vi "Update Block Status.vi"(4 "Writing":bool, 6 "Working":bool, 8 "Worker Error":errorcluster, 9 "Status In":T1={"State"=enum."Init", "i"=0, "Init"=FALSE, "Started"=FALSE, "Action"=enum."N/A"}, 11 "Status Queue In":refnum<queue>) -> (1 "Status":T1={"State"=enum."Init", "i"=0, "Init"=FALSE, "Started"=FALSE, "Action"=enum."N/A"}, 3 "Status Queue":refnum<queue>)   [LabVIEW 2020, in "FlexBlocks.lvlib"]
uses:
  FlexBlocks.lvlib
  Block Status.ctl
  Block State.ctl
  Run Action.ctl
  Block Status with Error.ctl
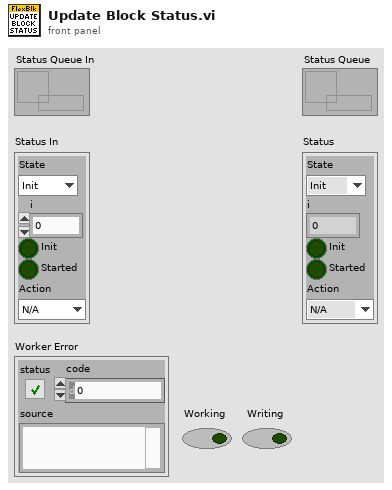
[diagram p1: front panel]
types:
  T1 = typedef "FlexBlocks.lvlib/Block Status.ctl" = cluster{"State":T2, "i":i32, "Init":bool, "Started":bool, "Action":T3}
  T2 = typedef "FlexBlocks.lvlib/Block State.ctl" = enum16{"Idle", "Init", "Start", "Run", "Stop"}
  T3 = typedef "FlexBlocks.lvlib/Run Action.ctl" = enum16{"N/A", "Read", "Work", "Write"}
  T4 = typedef "FlexBlocks.lvlib/Block Status with Error.ctl" = cluster{"Status":T1, "Error":errorcluster}
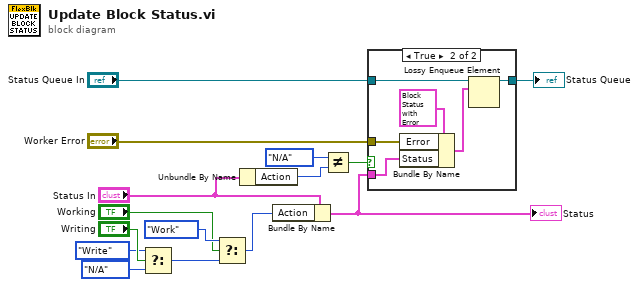
[diagram p0: block diagram]
diagram:
  n1 = Select(t=Run_Action."Write" ("Work Action"), s="Writing", f=Run_Action."N/A" ("Work Action")) -> (s? t:f=w11:T3)
  n2 = Select(t=Run_Action."Work" ("Work Action"), s="Working", f=w11) -> (s? t:f=w8:T3)
  n3 = Unbundle By Name("Status In") -> ("Action"=w6:T3)
  n4 = Bundle By Name(cluster="Status In", "Action"=w8) -> (w15:T1)
  "Status" <- w15
  n5 = Not Equal?(x=Run_Action."N/A", y=w6) -> (x != y?=w4:bool)
  n6 = case shown="True" w4 {
    tunnel: "Status Queue In" -> [w16 w22]
    tunnel: [w16 w21] -> w3
    tunnel: w15 -> [_ w17]
    tunnel: "Worker Error" -> [_ w18]
    frame False {
    }
    frame True {
      n7 = Bundle By Name(cluster=T4 {"Status"={"State"=enum."Init", "i"=0, "Init"=FALSE, "Started"=FALSE, "Action"=enum."N/A"}, "Error"={"status"=FALSE, "code"=0, "source"=""}} ("element"), "Error"=w18, "Status"=w17) -> (w19:T4)
      n8 = Lossy Enqueue Element(queue=w22, element=w19) -> (queue out=w21:refnum<queue>)  [unwired: 1 in, 3 out]
    }
  }
  "Status Queue" <- w3
